vi "Set Combobox Value.vi"(6 "Combo Box Ref":refnum<vi>, 7 "Data":path, 8 "error in (no error)":errorcluster, 9 "Run Mode?":bool, 10 "Indicator?":bool, 11 "Persistent Path Selector in":refnum<class "MGI Persistent Path Selector.lvclass">) -> (0 "error out":errorcluster, 3 "Persistent Path Selector out":refnum<class "MGI Persistent Path Selector.lvclass">)   [LabVIEW 2016, in "MGI Persistent Path Selector.lvclass"]
doc: "Updates the Combobox value to match the state of the XControl.\n\nAuthored by Shawn Walpole\nsupport@mooregoodideas.com\nwww.mooregoodideas.com\n\nCopyright (c) 2013, Moore Good Ideas, Inc.\n\nAll rights reserved.\n\nRedistribution and use in source and binary forms, with or without modification, are permitted provided that the following conditions are met:\n\n * Redistributions of source code must retain the above copyright notice, this list of conditions and the following disclaimer.\n * Redistributions in binary form must reproduce the above copyright notice, this list of conditions and the following disclaimer in the documentation and/or other materials provided with the distribution.\n * Neither the name of Moore Good Ideas, Inc. nor the names of its contributors may be used to endorse or promote products derived from this software without specific prior written permission.\n\nTHIS SOFTWARE IS PROVIDED BY THE COPYRIGHT HOLDERS AND CONTRIBUTORS \"AS IS\" AND ANY EXPRESS OR IMPLIED WARRANTIES, INCLUDING, BUT NOT LIMITED TO, THE IMPLIED WARRANTIES OF MERCHANTABILITY AND FITNESS FOR A PARTICULAR PURPOSE ARE DISCLAIMED. IN NO EVENT SHALL THE COPYRIGHT OWNER OR CONTRIBUTORS BE LIABLE FOR ANY DIRECT, INDIRECT, INCIDENTAL, SPECIAL, EXEMPLARY, OR CONSEQUENTIAL DAMAGES (INCLUDING, BUT NOT LIMITED TO, PROCUREMENT OF SUBSTITUTE GOODS OR SERVICES; LOSS OF USE, DATA, OR PROFITS; OR BUSINESS INTERRUPTION) HOWEVER CAUSED AND ON ANY THEORY OF LIABILITY, WHETHER IN CONTRACT, STRICT LIABILITY, OR TORT (INCLUDING NEGLIGENCE OR OTHERWISE) ARISING IN ANY WAY OUT OF THE USE OF THIS SOFTWARE, EVEN IF ADVISED OF THE POSSIBILITY OF SUCH DAMAGE."
uses:
  <userlib>/_MGI/User Interface/Path Selector XControl/Class Hierarchy/Persistent Path Selector/MGI Persistent Path Selector.lvclass
  <userlib>/_MGI/User Interface/Path Selector XControl/Class Hierarchy/Persistent Path Selector/MGI Persistent Path Selector.lvclass/MGI Persistent Path Selector.ctl
  <userlib>/_OpenG.lib/file/file.llb/Valid Path - Traditional__ogtk.vi
  <userlib>/_MGI/User Interface/Path Selector XControl/Class Hierarchy/MGI Path Selector.lvclass
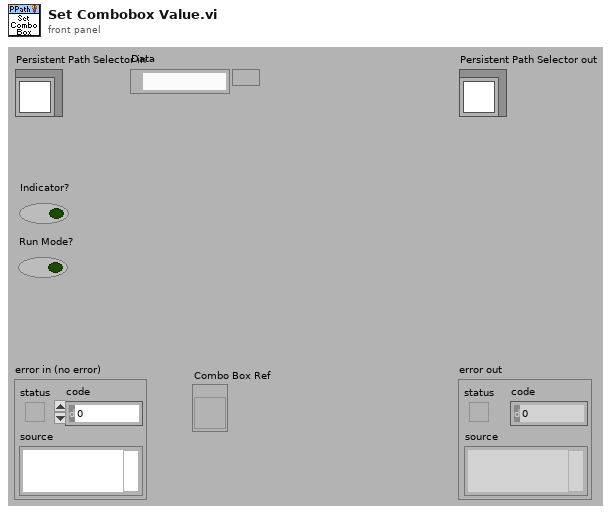
[diagram p1: front panel]
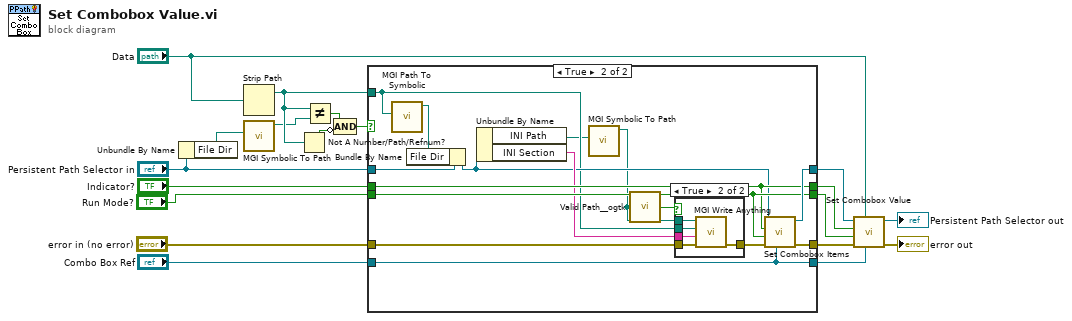
[diagram p0: block diagram]
diagram:
  n1 = Unbundle By Name("Persistent Path Selector in") -> ("File Dir"=w2:path)
  n2 = Strip Path(path="Data") -> (stripped path=w15:path)  [unwired: 1 out]
  n3 = call <userlib>:"MGI Symbolic To Path.vi"("Symbolic Path"=w2) -> ("Path"=w1:path)  [unwired: 8 in, 2 out]
  n4 = Not A Number/Path/Refnum?(number/path/refnum=w15) -> (NaN/Path/Refnum?=w17:bool)
  n5 = Not Equal?(x=w15, y=w1) -> (x != y?=w18:bool)
  n6 = Compound Arithmetic op=AND(w18, invert w17) -> (w16:bool)
  n7 = case shown="True" w16 {
    tunnel: w15 -> [_ w28]
    tunnel: "Persistent Path Selector in" -> [w22 w33]
    tunnel: "Indicator?" -> [w24 w35]
    tunnel: "Run Mode?" -> [w23 w36]
    tunnel: "Combo Box Ref" -> [w20 w39]
    tunnel: [w20 w39] -> w12
    tunnel: [w21 w38] -> w11
    tunnel: [w22 w37] -> w10
    tunnel: [w23 w36] -> w6
    tunnel: [w24 w35] -> w4
    tunnel: "error in (no error)" -> [w21 w31]
    frame False {
    }
    frame True {
      n8 = call <userlib>:"MGI Path To Symbolic.vi"("Path"=w28) -> ("Symbolic Path"=w27:path)  [unwired: 8 in, 2 out]
      n9 = Bundle By Name(cluster=w33, "File Dir"=w27) -> (w32:refnum<class "MGI Persistent Path Selector.lvclass">)
      n10 = Unbundle By Name(w32) -> ("INI Path"=w26:path, "INI Section"=w34:string)
      n11 = call <userlib>:"MGI Symbolic To Path.vi"("Symbolic Path"=w26) -> ("Path"=w25:path)  [unwired: 8 in, 2 out]
      n12 = call-poly <userlib>:"Valid Path__ogtk.vi"("path"=w25) -> ("valid"=w29:bool)
      n13 = case shown="True" w29 {
        tunnel: w34 -> [_ w45]
        tunnel: w25 -> [_ w44]
        tunnel: w31 -> [w40 w43]
        tunnel: [w40 w42] -> w30
        tunnel: w28 -> [_ w41]
        frame False {
        }
        frame True {
          n14 = call <userlib>:"MGI Write Anything.vi"("Error In"=w43, "Section Name (Name of \"Anything\")"=w45, "Anything"=w41, "Path (dialog)"=w44) -> ("Error Out"=w42:errorcluster)  [unwired: 5 in, 2 out]
        }
      }
      n15 = call-dynamic "Set Combobox Items.vi"("Combo Box Ref"=w39, "error in (no error)"=w30, "Run Mode?"=w36, "Indicator?"=w35, "Persistent Path Selector in"=w32) -> ("error out"=w38:errorcluster, "Persistent Path Selector out"=w37:refnum<class "MGI Persistent Path Selector.lvclass">)  [unwired: 4 in, 1 out]
    }
  }
  n16 = call-parent "Set Combobox Value.vi"("Combo Box Ref"=w12, "Data"="Data", "error in (no error)"=w11, "Run Mode?"=w6, "Indicator?"=w4, "Path Selector in"=w10) -> ("error out"=→"error out":errorcluster, "Path Selector out"=→"Persistent Path Selector out":refnum<class "MGI Persistent Path Selector.lvclass">)  [unwired: 4 in]
